vi "auto_turn.vi"(6 "direction":enum16{"right", "left"}(ring), 7 "timeout (ms)":dbl=-1.0, 8 "angle":dbl, 9 "speed":dbl, 10 "rightDrive":T2={"DeviceStatus"={"status"=FALSE, "code"=0, "source"=""}, "Type"=enum."PWM", "PWM"={"PWM Channel"=enum."Invalid", "DeadBand"={"Name"="", "maxPositivePwm"=0, "minPositivePwm"=0, "centerPwm"=0, "maxNegativePwm"=0, "minNegativePwm"=0, "angularRange"=0}}, "CAN"={"Device Number"=0, "SetOutput VI Ref"=variant(refnum<vi> refnum), "GetOutput VI Ref"=variant(refnum<vi> refnum), "Enable VI Ref"=variant(refnum<vi> refnum), "Disable VI Ref"=variant(refnum<vi> refnum), "Data"=variant}, "Invert"=FALSE, "DIO PWM"={"PWM \"Enable\" Channel"=enum."Invalid", "DIOChannel"=enum."Invalid", "PWM Rate"=0.0}}, 11 "leftDrive":T2={"DeviceStatus"={"status"=FALSE, "code"=0, "source"=""}, "Type"=enum."PWM", "PWM"={"PWM Channel"=enum."Invalid", "DeadBand"={"Name"="", "maxPositivePwm"=0, "minPositivePwm"=0, "centerPwm"=0, "maxNegativePwm"=0, "minNegativePwm"=0, "angularRange"=0}}, "CAN"={"Device Number"=0, "SetOutput VI Ref"=variant(refnum<vi> refnum), "GetOutput VI Ref"=variant(refnum<vi> refnum), "Enable VI Ref"=variant(refnum<vi> refnum), "Disable VI Ref"=variant(refnum<vi> refnum), "Data"=variant}, "Invert"=FALSE, "DIO PWM"={"PWM \"Enable\" Channel"=enum."Invalid", "DIOChannel"=enum."Invalid", "PWM Rate"=0.0}}) -> (2 "rightDrive":T2={"DeviceStatus"={"status"=FALSE, "code"=0, "source"=""}, "Type"=enum."PWM", "PWM"={"PWM Channel"=enum."Invalid", "DeadBand"={"Name"="", "maxPositivePwm"=0, "minPositivePwm"=0, "centerPwm"=0, "maxNegativePwm"=0, "minNegativePwm"=0, "angularRange"=0}}, "CAN"={"Device Number"=0, "SetOutput VI Ref"=variant(refnum<vi> refnum), "GetOutput VI Ref"=variant(refnum<vi> refnum), "Enable VI Ref"=variant(refnum<vi> refnum), "Disable VI Ref"=variant(refnum<vi> refnum), "Data"=variant}, "Invert"=FALSE, "DIO PWM"={"PWM \"Enable\" Channel"=enum."Invalid", "DIOChannel"=enum."Invalid", "PWM Rate"=0.0}}, 3 "leftDrive":T2={"DeviceStatus"={"status"=FALSE, "code"=0, "source"=""}, "Type"=enum."PWM", "PWM"={"PWM Channel"=enum."Invalid", "DeadBand"={"Name"="", "maxPositivePwm"=0, "minPositivePwm"=0, "centerPwm"=0, "maxNegativePwm"=0, "minNegativePwm"=0, "angularRange"=0}}, "CAN"={"Device Number"=0, "SetOutput VI Ref"=variant(refnum<vi> refnum), "GetOutput VI Ref"=variant(refnum<vi> refnum), "Enable VI Ref"=variant(refnum<vi> refnum), "Disable VI Ref"=variant(refnum<vi> refnum), "Data"=variant}, "Invert"=FALSE, "DIO PWM"={"PWM \"Enable\" Channel"=enum."Invalid", "DIOChannel"=enum."Invalid", "PWM Rate"=0.0}})   [LabVIEW 2017]
uses:
  <vilib>/Rock Robotics/WPI/MotorControl/WPI_MotorControlDeviceRef.ctl
  <vilib>/Rock Robotics/WPI/MotorControl/WPI_MotorControlType.ctl
  <vilib>/Rock Robotics/SystemInterfaces/DIO/FPGA_DIOPWMChannel.ctl
  <vilib>/Rock Robotics/WPI/PWM/WPI_PWMDeadband.ctl
  <vilib>/Rock Robotics/SystemInterfaces/DIO/FPGA_DIOChannel.ctl
  <vilib>/Rock Robotics/WPI/ThirdParty/Phoenix-LabVIEW/Motor Controller/Controls/CTRE_Phoenix_MotorControl_ControlMode.ctl
  <vilib>/Rock Robotics/Network Tables/NT Read Number.vi
  <vilib>/addons/control/pid/pid.llb/PID (DBL).vi
  <vilib>/addons/control/pid/NI_PID_pid.lvlib
panel:
  out "startYaw":dbl
  out "curYaw":dbl
  out "time":u32
  in  "posThresh":dbl=3.0 format="%#_13g"
  in  "velThresh":dbl=50.0 format="%#_13g"
  out "angle":dbl(graph)
  out "PID gains":T1={"proportional gain (Kc)"=200.0, "integral time (Ti, min)"=0.0, "derivative time (Td, min)"=0.001} {"derivative time (Td, min)" format="%.8f"; "integral time (Ti, min)" format="%.3f"; "proportional gain (Kc)" format="%.3f"}
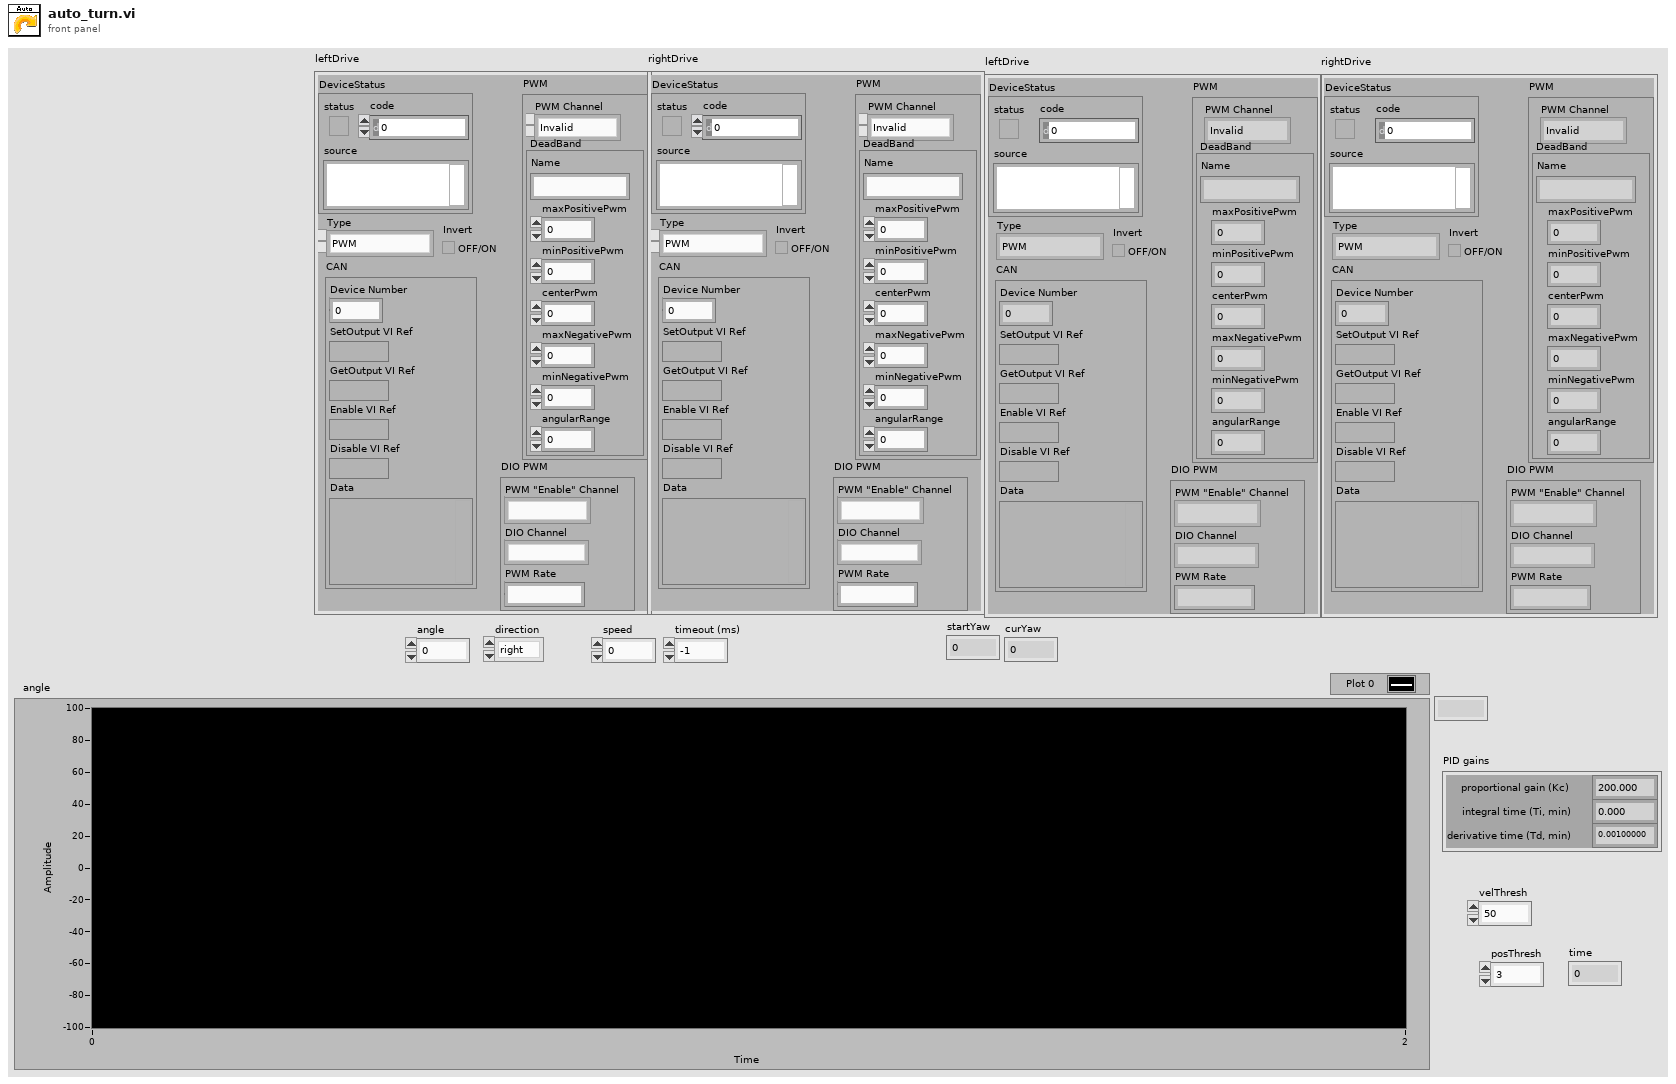
[diagram p1: front panel]
types:
  T1 = cluster{"proportional gain (Kc)":dbl, "integral time (Ti, min)":dbl, "derivative time (Td, min)":dbl}
  T2 = typedef "WPI_MotorControlDeviceRef.ctl" = cluster{"DeviceStatus":errorcluster, "Type":T3, "PWM":cluster{"PWM Channel":T4, "DeadBand":T5}, "CAN":cluster{"Device Number":u8, "SetOutput VI Ref":variant, "GetOutput VI Ref":variant, "Enable VI Ref":variant, "Disable VI Ref":variant, "Data":variant}, "Invert":bool, "DIO PWM":cluster{"PWM \"Enable\" Channel":T4, "DIOChannel":T6, "PWM Rate":dbl}}
  T3 = typedef "WPI_MotorControlType.ctl" = enum16{"PWM", "CAN", "DIO PWM"}
  T4 = typedef "FPGA_DIOPWMChannel.ctl" = enum8{"PWM 0", "PWM 1", "PWM 2", "PWM 3", "PWM 4", "PWM 5", "PWM 6", "PWM 7", "PWM 8", "PWM 9", "PWM MXP 0", "PWM MXP 1", "PWM MXP 2", "PWM MXP 3", "PWM MXP 4", "PWM MXP 5", "PWM MXP 6", "PWM MXP 7", "PWM MXP 8", "PWM MXP 9", "Invalid"}
  T5 = typedef "WPI_PWMDeadband.ctl" = cluster{"Name":string, "maxPositivePwm":i32, "minPositivePwm":i32, "centerPwm":i32, "maxNegativePwm":i32, "minNegativePwm":i32, "angularRange":u16}
  T6 = typedef "FPGA_DIOChannel.ctl" = enum8{"DIO 0", "DIO 1", "DIO 2", "DIO 3", "DIO 4", "DIO 5", "DIO 6", "DIO 7", "DIO 8", "DIO 9", "DIO MXP 0", "DIO MXP 1", "DIO MXP 2", "DIO MXP 3", "DIO MXP 4", "DIO MXP 5", "DIO MXP 6", "DIO MXP 7", "DIO MXP 8", "DIO MXP 9", "DIO MXP 10", "DIO MXP 11", "DIO MXP 12", "DIO MXP 13", "DIO MXP 14", "DIO MXP 15", "SPI Port CS1", "SPI Port CS2", "SPI Port CS3", "SPI Port MISO", "SPI Port MOSI", "Invalid"}
  T7 = typedef "CTRE_Phoenix_MotorControl_ControlMode.ctl" = u16
  T8 = cluster{"Numeric":dbl, "Numeric":dbl, "Numeric":dbl}
  T9 = cluster{"Rollover":dbl, "Yaw":dbl, "Cont Yaw":dbl}
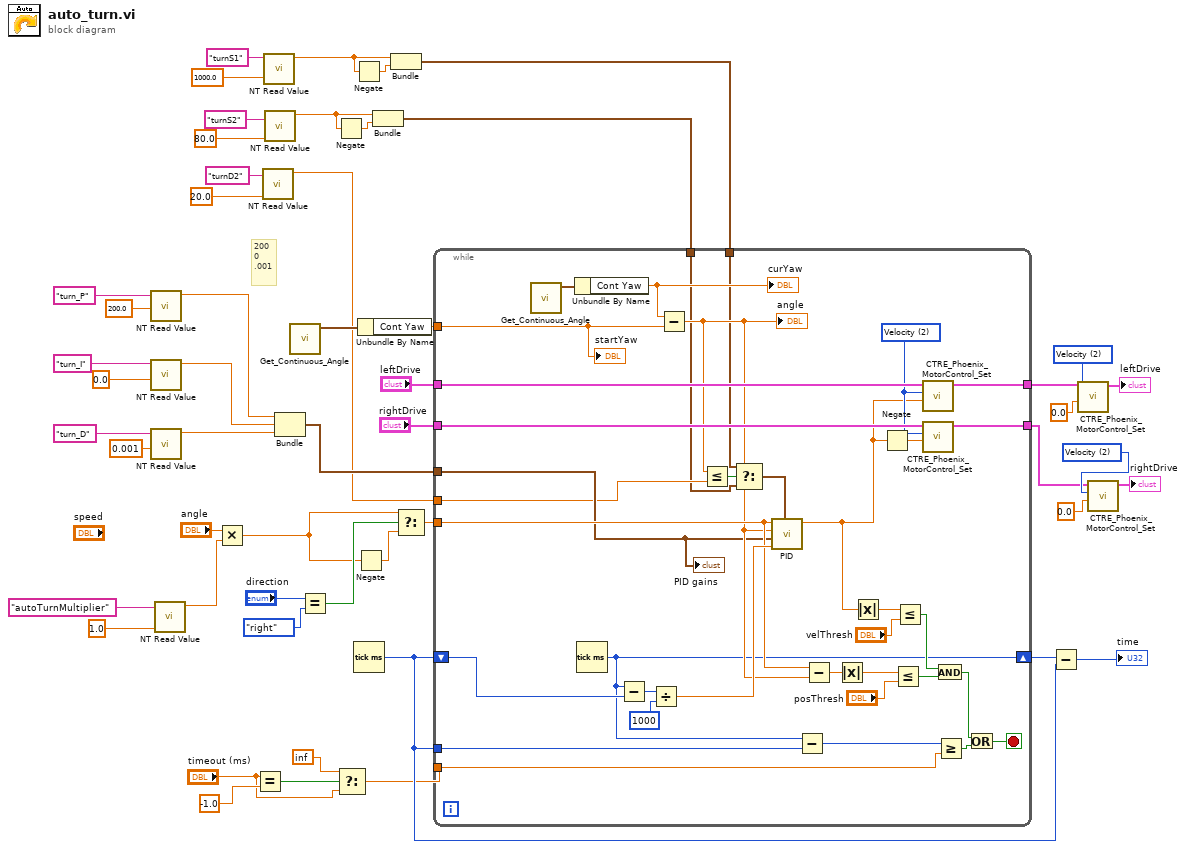
[diagram p0: block diagram]
diagram:
  w47 = T7 2 items=["PercentOutput"=0, "Position"=1, "Velocity"=2, "Current"=3, "Follower"=5, "MotionProfile"=6, "MotionMagic"=7, "MotionMagicArc"=8, "MotionProfileArc"=10, "Disabled"=15] ("Control Mode")
  w48 = T7 2 items=["PercentOutput"=0, "Position"=1, "Velocity"=2, "Current"=3, "Follower"=5, "MotionProfile"=6, "MotionMagic"=7, "MotionMagicArc"=8, "MotionProfileArc"=10, "Disabled"=15] ("Control Mode")
  # "200\n0\n.001"
  n1 = call-poly <vilib>:"NT Read Value.vi"("Default Value"=200.0, "Name"="turn_P") -> ("Numeric"=w17:dbl)  [unwired: 8 in, 1 out]
  n2 = call-poly <vilib>:"NT Read Value.vi"("Default Value"=0.0, "Name"="turn_I") -> ("Numeric"=w16:dbl)  [unwired: 8 in, 1 out]
  n3 = call-poly <vilib>:"NT Read Value.vi"("Default Value"=0.001, "Name"="turn_D") -> ("Numeric"=w15:dbl)  [unwired: 8 in, 1 out]
  n4 = call-poly <vilib>:"NT Read Value.vi"("Default Value"=1.0, "Name"="autoTurnMultiplier") -> ("Numeric"=w35:dbl)  [unwired: 8 in, 1 out]
  n5 = Multiply(x="angle", y=w35) -> (x*y=w36:dbl)
  n6 = Equal?(x="timeout (ms)", y=-1.0) -> (x = y?=w27:bool)
  n7 = call-poly <vilib>:"NT Read Value.vi"("Default Value"=20.0, "Name"="turnD2") -> ("Numeric"=w7:dbl)  [unwired: 8 in, 1 out]
  n8 = call-poly <vilib>:"NT Read Value.vi"("Default Value"=1000.0, "Name"="turnS1") -> ("Numeric"=w5:dbl)  [unwired: 8 in, 1 out]
  n9 = call-poly <vilib>:"NT Read Value.vi"("Default Value"=80.0, "Name"="turnS2") -> ("Numeric"=w2:dbl)  [unwired: 8 in, 1 out]
  n10 = Bundle("Numeric"=w17, "Numeric"=w16, "Numeric"=w15) -> (w14:T8)  [unwired: 1 in]
  n11 = call <vilib>:"Get_Continuous_Angle.vi"() -> ("Continuous Angle"=w44:T9)  [unwired: 11 in]
  n12 = Equal?(x="direction", y=enum16{"right", "left"}."right") -> (x = y?=w43:bool)
  n13 = Negate(x=w2) -> (-x=w3:dbl)
  n14 = Select(t=inf, s=w27, f="timeout (ms)") -> (s? t:f=w24:dbl)
  n15 = Negate(x=w5) -> (-x=w6:dbl)
  n16 = Tick Count (ms)() -> (millisecond timer value=w29:u32)
  n17 = Negate(x=w36) -> (-x=w42:dbl)
  n18 = Unbundle By Name(w44) -> ("Cont Yaw"=w53:dbl)
  n19 = Bundle("Numeric"=w2, w3) -> (w1:cluster{"Numeric":dbl, dbl})  [unwired: 1 in]
  n20 = Bundle("Numeric"=w5, w6) -> (w4:cluster{"Numeric":dbl, dbl})  [unwired: 1 in]
  n21 = Select(t=w36, s=w43, f=w42) -> (s? t:f=w30:dbl)
  n22 = while {
    tunnel: w53 -> [w58]
    shift-right: [w62] -> w32
    shift-left: w29 -> [w87]
    tunnel: w30 -> [w72]
    tunnel: "leftDrive" -> [w83]
    tunnel: "rightDrive" -> [w82]
    tunnel: [w79] -> w39
    tunnel: [w78] -> w38
    tunnel: w29 -> [w61]
    tunnel: w24 -> [w59]
    tunnel: w14 -> [w57]
    tunnel: w7 -> [w56]
    tunnel: w4 -> [w55]
    tunnel: w1 -> [w54]
    stop <- w65 stop-if-true
    w80 = T7 2 items=["PercentOutput"=0, "Position"=1, "Velocity"=2, "Current"=3, "Follower"=5, "MotionProfile"=6, "MotionMagic"=7, "MotionMagicArc"=8, "MotionProfileArc"=10, "Disabled"=15] ("Control Mode")
    n23 = call <vilib>:"Get_Continuous_Angle.vi"() -> ("Continuous Angle"=w89:T9)  [unwired: 11 in]
    n24 = Unbundle By Name(w89) -> ("Cont Yaw"=w88:dbl)
    "curYaw" <- w88
    n25 = Tick Count (ms)() -> (millisecond timer value=w62:u32)
    n26 = Subtract(x=w62, y=w87) -> (x-y=w86:u32)
    n27 = Divide(x=w86, y=u32 1000) -> (x/y=w85:dbl)
    n28 = Subtract(x=w88, y=w58) -> (x-y=w66:dbl)
    "angle" <- w66
    n29 = Less Or Equal?(x=w66, y=w56) -> (x <= y?=w67:bool)
    n30 = Select(t=w55, s=w67, f=w54) -> (s? t:f=w68:cluster{"Numeric":dbl, dbl})
    n31 = call-poly <vilib>:"PID.vi"("output range"=w68, "dt (s)"=w85, "PID gains"=w57, "process variable"=w66, "setpoint"=w72) -> ("output"=w75:dbl)  [unwired: 5 in, 1 out]
    n32 = Subtract(x=w62, y=w61) -> (x-y=w60:u32)
    n33 = Subtract(x=w72, y=w66) -> (x-y=w71:dbl)
    n34 = Absolute Value(x=w71) -> (abs(x)=w70:dbl)
    n35 = Absolute Value(x=w75) -> (abs(x)=w74:dbl)
    n36 = Negate(x=w75) -> (-x=w81:dbl)
    n37 = Less Or Equal?(x=w70, y="posThresh") -> (x <= y?=w77:bool)
    n38 = Less Or Equal?(x=w74, y="velThresh") -> (x <= y?=w76:bool)
    n39 = call <vilib>:"CTRE_Phoenix_MotorControl_Set.vi"("Output"=w75, "Control Mode"=w80, "PhoenixMotorControlDevRef"=w83) -> ("PhoenixMotorControlDevRef"=w79:T2)  [unwired: 7 in, 1 out]
    n40 = call <vilib>:"CTRE_Phoenix_MotorControl_Set.vi"("Output"=w81, "Control Mode"=w80, "PhoenixMotorControlDevRef"=w82) -> ("PhoenixMotorControlDevRef"=w78:T2)  [unwired: 7 in, 1 out]
    n41 = And(x=w76, y=w77) -> (x .and. y?=w64:bool)
    n42 = Greater Or Equal?(x=w60, y=w59) -> (x >= y?=w63:bool)
    n43 = Or(x=w64, y=w63) -> (x .or. y?=w65:bool)
    "PID gains" <- w57
    "startYaw" <- w58
  }
  n44 = Subtract(x=w32, y=w29) -> (x-y=→"time":u32)
  n45 = call <vilib>:"CTRE_Phoenix_MotorControl_Set.vi"("Output"=0.0, "Control Mode"=w47, "PhoenixMotorControlDevRef"=w39) -> ("PhoenixMotorControlDevRef"=→"leftDrive":T2)  [unwired: 7 in, 1 out]
  n46 = call <vilib>:"CTRE_Phoenix_MotorControl_Set.vi"("Output"=0.0, "Control Mode"=w48, "PhoenixMotorControlDevRef"=w38) -> ("PhoenixMotorControlDevRef"=→"rightDrive":T2)  [unwired: 7 in, 1 out]
